vi "Execute Default Event.vi"(10 "Command":string, 11 "Library in":refnum<vi>) -> (0 "error out":errorcluster)   [LabVIEW 2020, in "Panter Dashboard.lvlib"]
uses:
  Panter Dashboard.lvlib
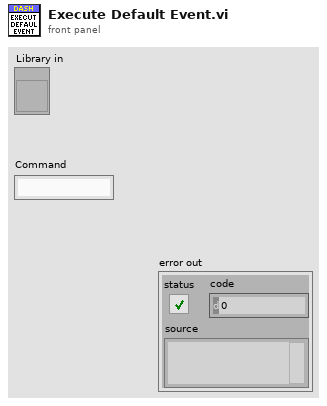
[diagram p1: front panel]
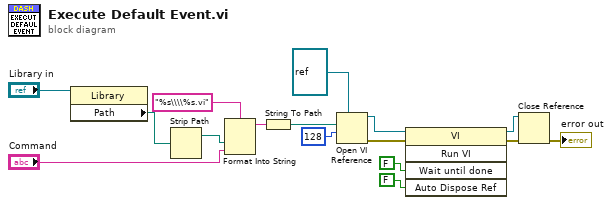
[diagram p0: block diagram]
diagram:
  n1 = property class="Library"(reference="Library in") -> ("Path"=w3:path)  [unwired: 1 in, 2 out]
  n2 = Strip Path(path=w3) -> (stripped path=w2:path)  [unwired: 1 out]
  n3 = Format Into String(format string="%s\\\\%s.vi", w2, "Command") -> (resulting string=w6:string)  [unwired: 2 in, 1 out]
  n4 = String To Path(string=w6) -> (path=w5:path)
  n5 = Open VI Reference(type specifier VI Refnum (for type only)=refnum<vi> refnum, vi path=w5, options=128) -> (vi reference=w8:refnum<vi>, error out=w16:errorcluster)  [unwired: 3 in]
  n6 = invoke class="VI" method="Run VI"(reference=w8, error in=w16, "Wait until done"=FALSE ("Wait Until Done"), "Auto Dispose Ref"=FALSE ("Auto Dispose Reference")) -> (reference out=w7:refnum<vi>, error out=w15:errorcluster)  [unwired: 1 in, 3 out]
  n7 = Close Reference(reference=w7, error in (no error)=w15) -> (error out=→"error out":errorcluster)
